vi "splitter position calc.vi"(8 "ExpandSize":i32, 9 "CollapseDirection":T1, 10 "Splitter":refnum<vi>, 11 "Front Panel":refnum<vi>) -> (0 "Splitter Position":i32, 2 "Splitter":refnum<vi>, 3 "Front Panel":refnum<vi>)   [LabVIEW 2021, in "CollapsePanel.lvclass"]
uses:
  CollapsePanel.lvclass
  collapse direction.ctl
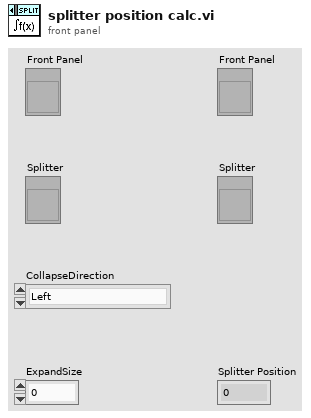
[diagram p1: front panel]
types:
  T1 = typedef "CollapsePanel.lvclass/collapse direction.ctl" = enum16{"Left", "Right", "Up", "Down"}
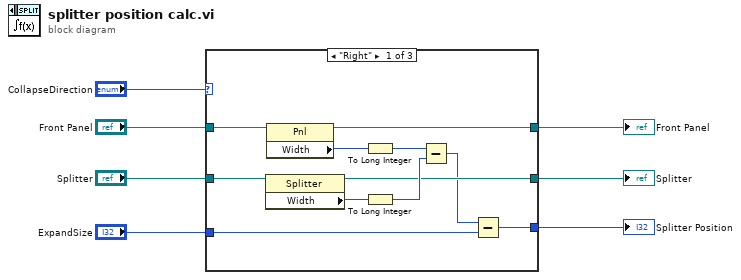
[diagram p0: block diagram]
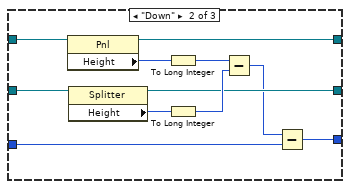
[diagram p2: hidden frame]
diagram:
  n1 = case shown="\"Right\"" "CollapseDirection" {
    tunnel: "Front Panel" -> [w18 w29 w32]
    tunnel: "Splitter" -> [w17 w28 w31]
    tunnel: [w8 w19 w30] -> w1
    tunnel: [w12 w22 w32] -> w5
    tunnel: [w11 w23 w31] -> w4
    tunnel: "ExpandSize" -> [w9 w20 w30]
    frame "Right" {
      n2 = property class="Splitter"(reference=w17) -> (reference out=w11:refnum<vi>, "Width"=w15:u32)  [unwired: 1 in, 1 out]
      n3 = property class="Pnl"(reference=w18) -> (reference out=w12:refnum<vi>, "Width"=w16:u32)  [unwired: 1 in, 1 out]
      n4 = To Long Integer(number=w16) -> (32bit integer=w13:i32)
      n5 = To Long Integer(number=w15) -> (32bit integer=w14:i32)
      n6 = Subtract(x=w13, y=w14) -> (x-y=w10:i32)
      n7 = Subtract(x=w10, y=w9) -> (x-y=w8:i32)
    }
    frame "Down" {
      n8 = property class="Pnl"(reference=w29) -> (reference out=w22:refnum<vi>, "Height"=w27:u32)  [unwired: 1 in, 1 out]
      n9 = property class="Splitter"(reference=w28) -> (reference out=w23:refnum<vi>, "Height"=w26:u32)  [unwired: 1 in, 1 out]
      n10 = To Long Integer(number=w27) -> (32bit integer=w24:i32)
      n11 = To Long Integer(number=w26) -> (32bit integer=w25:i32)
      n12 = Subtract(x=w24, y=w25) -> (x-y=w21:i32)
      n13 = Subtract(x=w21, y=w20) -> (x-y=w19:i32)
    }
    frame "Left", "Up" {
    }
  }
  "Front Panel" <- w5
  "Splitter" <- w4
  "Splitter Position" <- w1
